vi "Run Test (Object Array).vi"(5 "Test Report":refnum<class "Test Report.lvclass">, 6 "Verbose":bool, 7 "Report Path":path, 8 "error in":errorcluster, 10 "Objects":refnum<class>[](array[class]), 11 "Interactive (T)":bool=TRUE) -> (0 "error out":errorcluster)   [LabVIEW 2013, in "Caraya.lvlib"]
uses:
  Caraya.lvlib
  classes/Test Report/Test Report.lvclass
  classes/Test Runner.Class/Test Runner.Class.lvclass
  classes/Test Runner/Test Runner.lvclass
  classes/Test Runner.Collection/Test Runner.Collection.lvclass
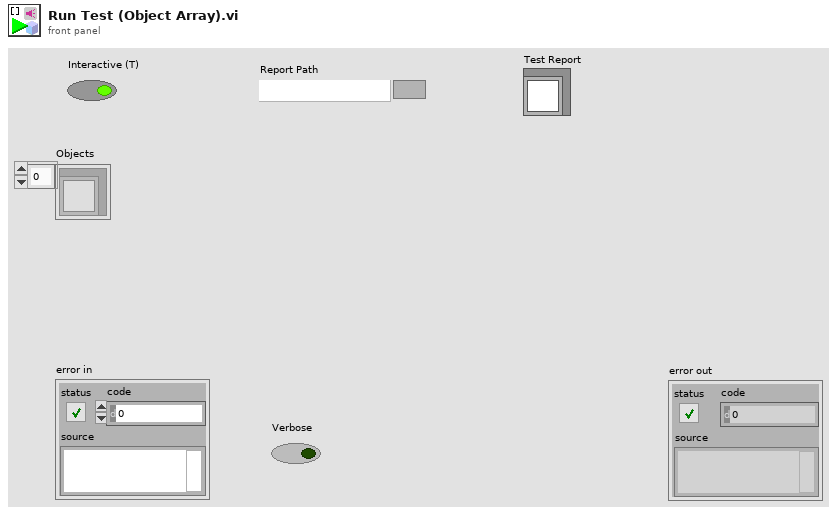
[diagram p1: front panel]
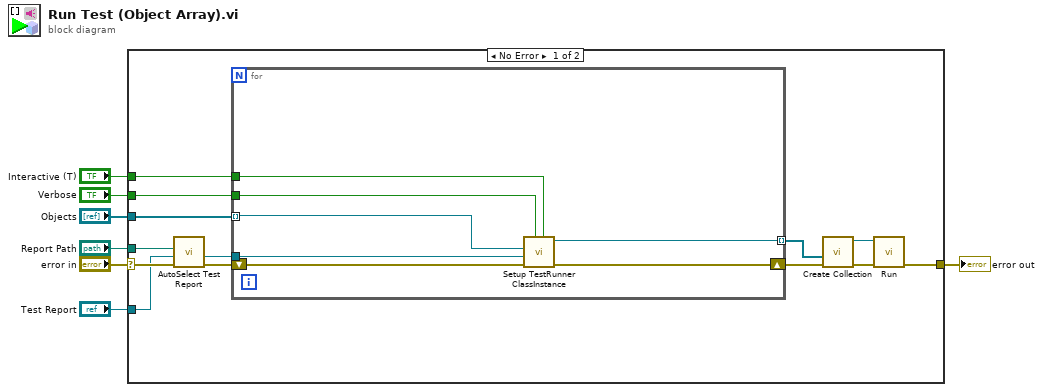
[diagram p0: block diagram]
diagram:
  n1 = case shown="No Error" "error in" {
    selector: "error in" -> [w17 w28]
    tunnel: [w20 w28] -> w7
    tunnel: "Verbose" -> [w19 _]
    tunnel: "Interactive (T)" -> [w18 _]
    tunnel: "Test Report" -> [w15 _]
    tunnel: "Objects" -> [w14 _]
    tunnel: "Report Path" -> [w16 _]
    frame No Error {
      n2 = call "AutoSelect Test Report.vi"("error in (no error)"=w17, "Test Report in"=w15, "Report Path"=w16) -> ("error out"=w13:errorcluster, "Test Report out"=w8:refnum<class "Test Report.lvclass">)  [unwired: 7 in]
      n3 = for {
        tunnel: w19 -> [w27]
        tunnel: w18 -> [w26]
        tunnel: w14 -> [w23] mode=indexing
        tunnel: [w22] -> w12 mode=indexing
        shift-right: [w21] -> w11
        shift-left: w13 -> [w24]
        tunnel: w8 -> [w25]
        n4 = call "Setup TestRunner ClassInstance.vi"("Interactive (T)"=w26, "Verbose (F)"=w27, "error in (no error)"=w24, "Test Report"=w25, "Instance"=w23) -> ("error out"=w21:errorcluster, "Test Runner.Class out"=w22:refnum<class "Test Runner.Class.lvclass">)  [unwired: 5 in]
      }
      n5 = call "Create Collection.vi"("error in (no error)"=w11, "Test Runners"=w12) -> ("error out"=w10:errorcluster, "Test Runner.Collection out"=w9:refnum<class "Test Runner.Collection.lvclass">)  [unwired: 8 in]
      n6 = call "Run.vi"("error in (no error)"=w10, "Test Runner in"=w9) -> ("error out"=w20:errorcluster)  [unwired: 8 in, 1 out]
    }
    frame Error {
    }
  }
  "error out" <- w7
